vi "Send command.vi"(8 "error in (no error)":errorcluster, 10 "message":string, 11 "SIM_Roda_Filtros in":refnum<class "SIM_Roda_Filtros.lvclass">) -> (0 "error out":errorcluster, 3 "SIM_Roda_Filtros out":refnum<class "SIM_Roda_Filtros.lvclass">)   [LabVIEW 2018, in "SIM_Roda_Filtros.lvclass"]
uses:
  SIM_Roda_Filtros.lvclass
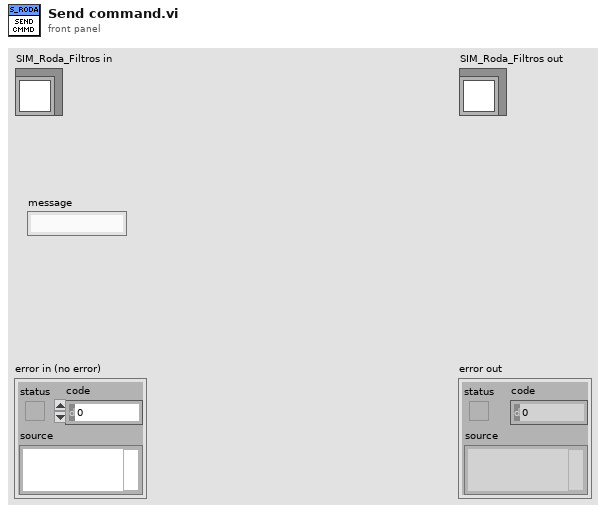
[diagram p1: front panel]
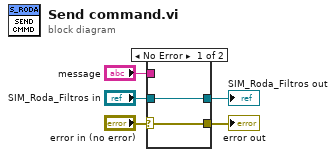
[diagram p0: block diagram]
diagram:
  n1 = case shown="No Error" "error in (no error)" {
    selector: "error in (no error)" -> [w7 w8]
    tunnel: [w7 w8] -> w4
    tunnel: "SIM_Roda_Filtros in" -> [w6 w9]
    tunnel: [w6 w9] -> w2
    tunnel: "message" -> [_ _]
    frame No Error {
    }
    frame Error {
    }
  }
  "error out" <- w4
  "SIM_Roda_Filtros out" <- w2
